vi "PID Circular Buffer.vi"(5 "initialize":bool, 10 "sample length":i32=100, 11 "input data point":dbl format="%0.2f") -> (0 "error":i32, 3 "Current Queue":dbl[](array[numeric]))   [LabVIEW 2020, in "NI_PID_autopid.lvlib"]
uses:
  <vilib>/addons/control/pid/NI_PID_autopid.lvlib
panel:
  out "current length":i32
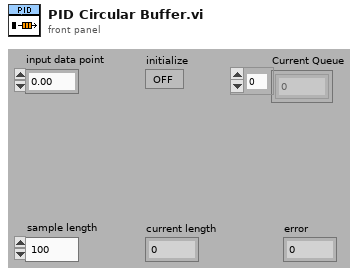
[diagram p1: front panel]
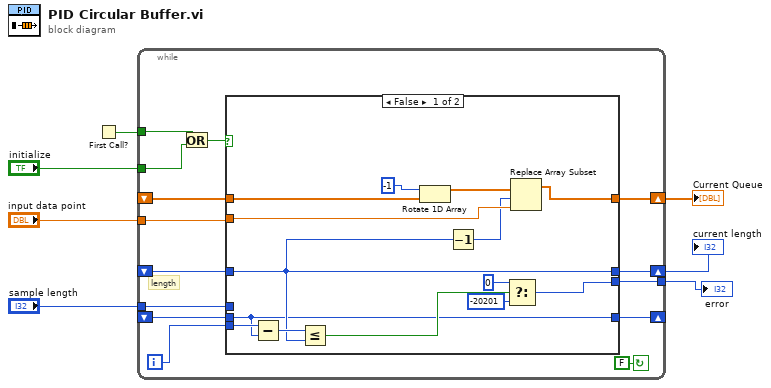
[diagram p0: block diagram]
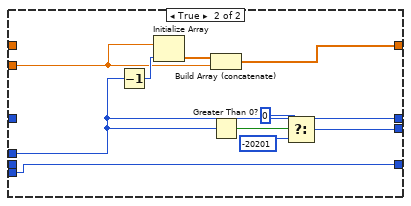
[diagram p2: hidden frame]
diagram:
  n1 = First Call?() -> (First Call?: T/F=w5:bool)
  n2 = while {
    tunnel: w5 -> [w16]
    shift-left: _ -> [w19]
    shift-right: [w20] -> w6
    shift-left: _ -> [w18]
    shift-right: [w21] -> w7
    tunnel: "input data point" -> [w14]
    tunnel: "initialize" -> [w13]
    tunnel: "sample length" -> [w12]
    shift-right: [w10] -> _
    shift-left: _ -> [w9]
    tunnel: [w8] -> w1
    i -> [w11]
    stop <- FALSE continue-if-true
    # "length"
    n3 = Or(x=w16, y=w13) -> (x .or. y?=w15:bool)
    n4 = case shown="False" w15 {
      tunnel: [w33 w43] -> w21
      tunnel: [w30 w38] -> w20
      tunnel: w19 -> [w30 _]
      tunnel: w18 -> [w34 _]
      tunnel: w14 -> [w35 w39]
      tunnel: w12 -> [_ w38]
      tunnel: w11 -> [w32 w37]
      tunnel: [w25 w37] -> w10
      tunnel: w9 -> [w25 _]
      tunnel: [w26 w36] -> w8
      frame False {
        n5 = Subtract(x=w32, y=w25) -> (x-y=w31:i32)
        n6 = Less Or Equal?(x=w31, y=w30) -> (x <= y?=w27:bool)
        n7 = Rotate 1D Array(1:w34, 2:i16 -1 ("n")) -> (0:w22:dbl[])
        n8 = Decrement(x=w30) -> (x-1=w23:i32)
        n9 = Select(t=0, s=w27, f=-20201) -> (s? t:f=w26:i32)
        n10 = Replace Array Subset(array=w22, new element=w35, index=w23) -> (w33:dbl[])
      }
      frame True {
        n11 = Decrement(x=w38) -> (x-1=w45:i32)
        n12 = Initialize Array(w39, w45) -> (w44:dbl[])
        n13 = Build Array (concatenate)(w44, w39) -> (w43:dbl[])
        n14 = Greater Than 0?(x=w38) -> (x > 0?=w42:bool)
        n15 = Select(t=0, s=w42, f=-20201) -> (s? t:f=w36:i32)
      }
    }
  }
  "Current Queue" <- w7
  "current length" <- w6
  "error" <- w1
